vi "Ctor.vi"(8 "error in (no error)":errorcluster, 10 "Panel Ref":refnum<vi>, 11 "List Ref":refnum<vi>) -> (0 "error out":errorcluster, 3 "BetterSearch out":refnum<class "BetterSearch.lvclass">)   [LabVIEW 2020, in "Better Search.lvlib" / "BetterSearch.lvclass"]
uses:
  BetterSearch.lvclass
  Data Types/Search Params.ctl
  Data Types/Search Type.ctl
  Data Types/Search Scope.ctl
  Data Types/Scope Options.ctl
  BetterSearch.lvclass/BetterSearch.ctl
  Better Search.lvlib
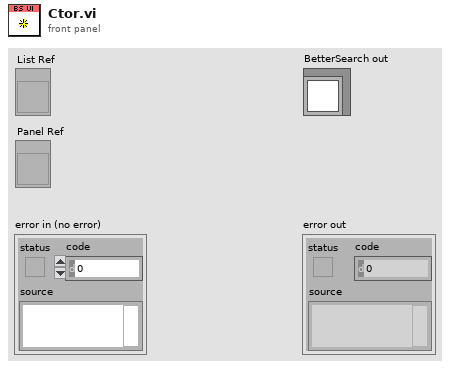
[diagram p1: front panel]
types:
  T1 = typedef "Better Search.lvlib/Search Params.ctl" = cluster{"Type":T2, "Type ID":string, "Text":string, "Scope":T3, "Targets":refnum<vi>[], "Scope Options":T4, "Typedef Path":path, "Member Graph Index":i32, "Member TypeID":string}
  T2 = typedef "Better Search.lvlib/Search Type.ctl" = enum16{"Generic", "Text", "Data Type", "VI", "Node"}
  T3 = typedef "Better Search.lvlib/Search Scope.ctl" = enum16{"Active Target", "Active Project", "Specific Targets", "Active VI", "Active Hierarchy"}
  T4 = typedef "Better Search.lvlib/Scope Options.ctl" = cluster{"Include Labels":bool, "Include Captions":bool, "Include Node Name":bool, "Member Access":bool, "Member Read":bool, "Member Write":bool, "Member Name":string, "String Value":bool, "Dependencies":bool, "vi.lib":bool, "user.lib":bool, "instr.lib":bool}
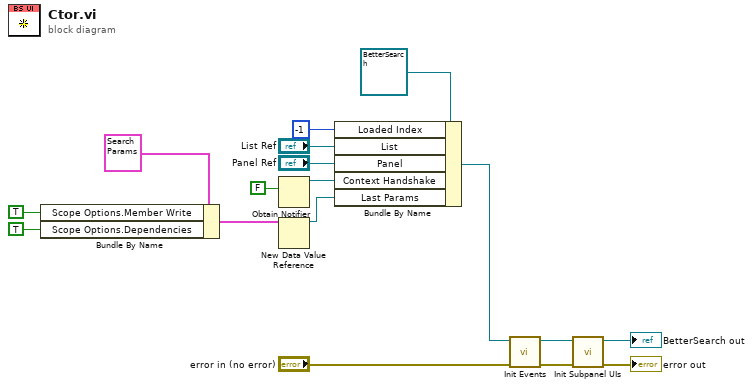
[diagram p0: block diagram]
diagram:
  n1 = Bundle By Name(cluster=T1 {"Type"=enum."Generic", "Type ID"="", "Text"="", "Scope"=enum."Active Target", "Targets"=[], "Scope Options"={"Include Labels"=FALSE, "Include Captions"=FALSE, "Include Node Name"=FALSE, "Member Access"=FALSE, "Member Read"=FALSE, "Member Write"=FALSE, "Member Name"="", "String Value"=FALSE, "Dependencies"=FALSE, "vi.lib"=FALSE, "user.lib"=FALSE, "instr.lib"=FALSE}, "Typedef Path"=path "", "Member Graph Index"=0, "Member TypeID"=""} ("Search Params"), "Scope Options.Member Write"=TRUE, "Scope Options.Dependencies"=TRUE) -> (w4:T1)
  n2 = Obtain Notifier(notification data type=FALSE) -> (notifier out=w7:refnum<notifier>)  [unwired: 3 in, 2 out]
  n3 = New Data Value Reference(data value=w4) -> (data value reference=w5:refnum<data-value>)  [unwired: 1 in, 1 out]
  n4 = Bundle By Name(cluster=refnum<class "BetterSearch.lvclass"> refnum ("BetterSearch in"), "Loaded Index"=-1, "List"="List Ref", "Panel"="Panel Ref", "Context Handshake"=w7, "Last Params"=w5) -> (w14:refnum<class "BetterSearch.lvclass">)
  n5 = call "Init Events.vi"("error in (no error)"="error in (no error)", "BetterSearch in"=w14) -> ("error out"=w11:errorcluster, "BetterSearch out"=w12:refnum<class "BetterSearch.lvclass">)  [unwired: 8 in]
  n6 = call "Init Subpanel UIs.vi"("error in (no error)"=w11, "BetterSearch in"=w12) -> ("error out"=→"error out":errorcluster, "BetterSearch out"=→"BetterSearch out":refnum<class "BetterSearch.lvclass">)  [unwired: 8 in]
